vi "main.vi"() -> ()   [LabVIEW 2023]
uses:
  Controls/insutrument_data.ctl
  Controls/table_data.ctl
  <vilib>/Utility/error.llb/DialogType.ctl
  Controls/errors_type.ctl
panel:
  out "Description":string
  out "Time":string
  out "Error Code":string
  out "Type":T1
  out "Table 2":string[][](table)
  in  "stop 2":bool
  out "Waveform Chart 2":i32(graph)
  out "PSRR (dB) 2":i32
  in  "Eror log":bool
  out "Error?":bool
  in  "Wait time (sec)":i32=1 step=1
  out "error out":errorcluster
  in  "error in":errorcluster
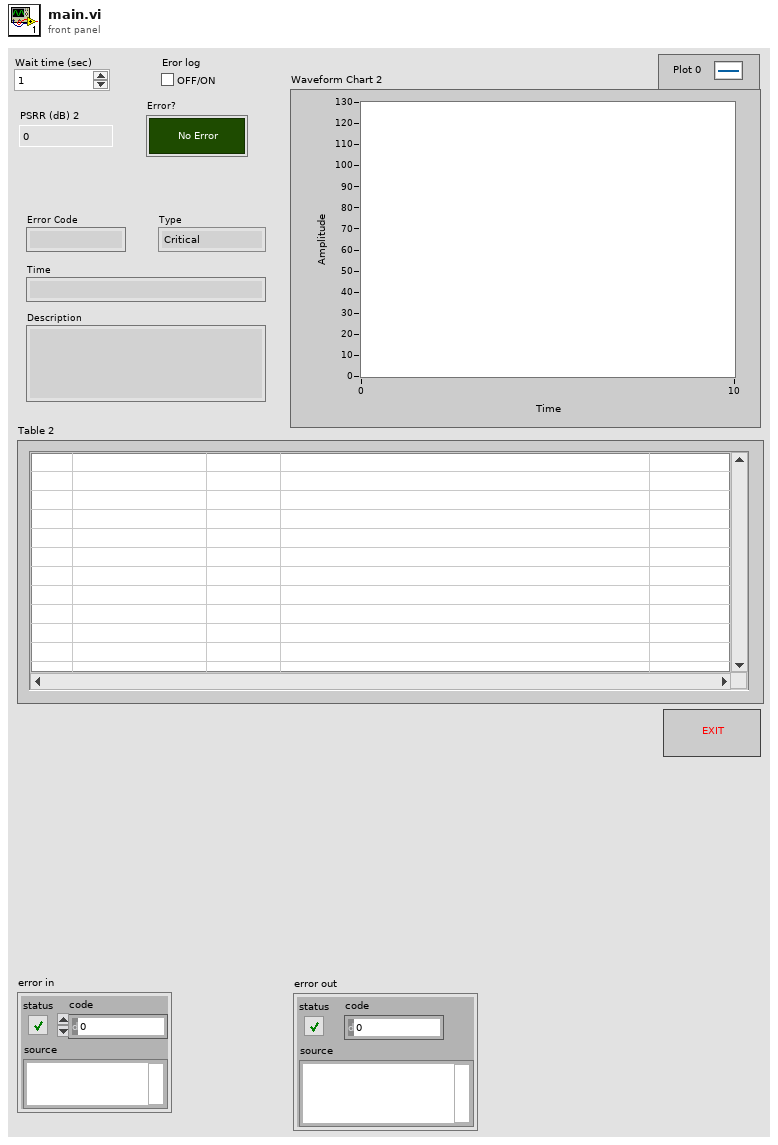
[diagram p1: front panel]
types:
  T1 = typedef "errors_type.ctl" = enum16{"Critical", "No error", "Warning", "Passive", "Unknown"}
  T2 = typedef "table_data.ctl" = cluster{"Passive_err":i32, "Unkown_err":i32, "Table_data":T3[][], "Err_log_sn":i32}
  T3 = typedef "insutrument_data.ctl" = string
  T4 = cluster{"Error Code":string, "Time":string, "Description":string, "Type":T1}
  T5 = typedef "DialogType.ctl" = u16
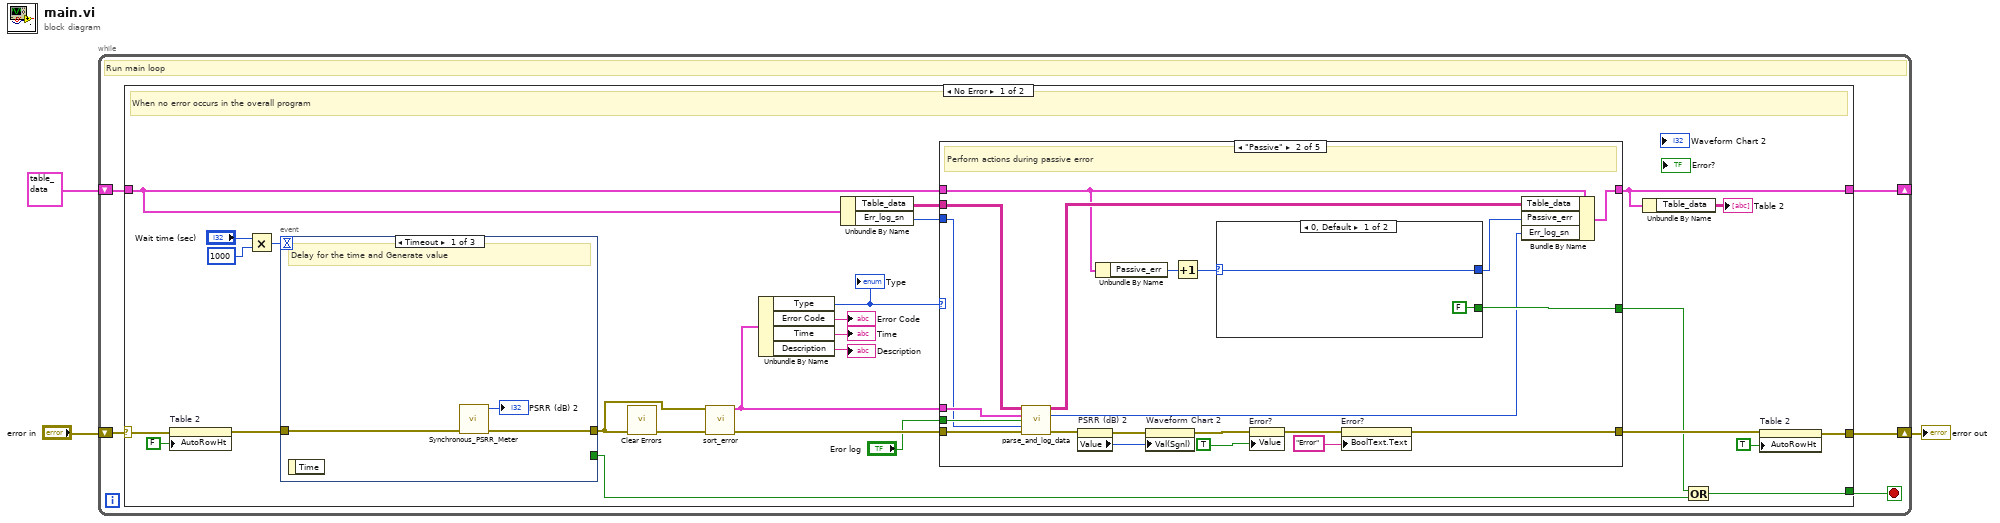
[diagram p0: block diagram]
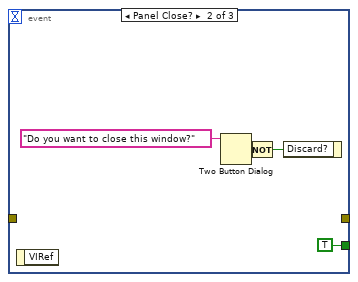
[diagram p2: hidden frame]
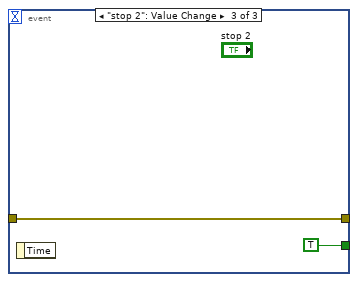
[diagram p3: hidden frame]
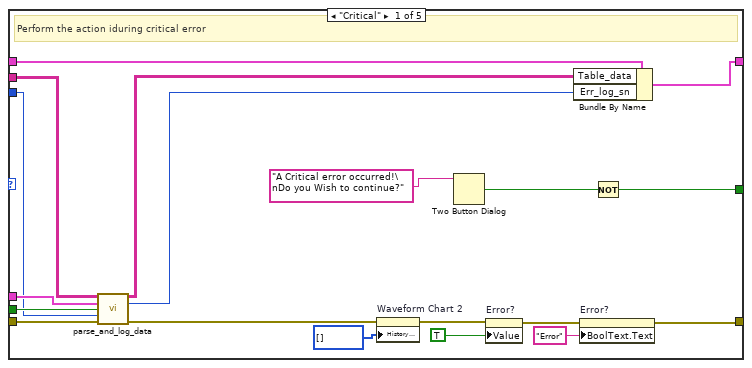
[diagram p4: hidden frame]
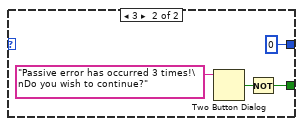
[diagram p5: hidden frame]
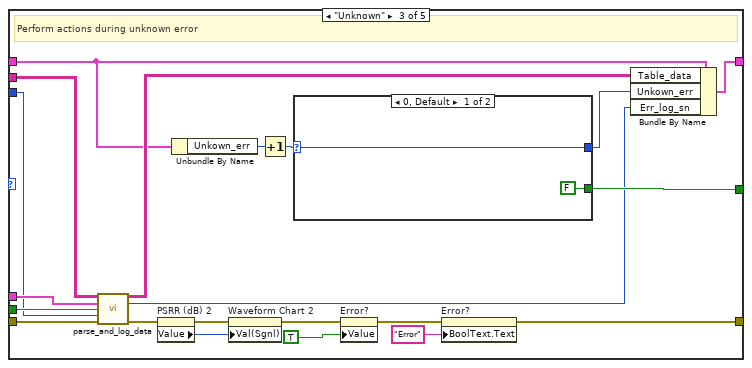
[diagram p6: hidden frame]
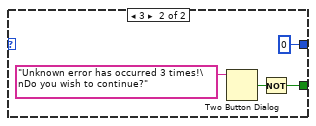
[diagram p7: hidden frame]
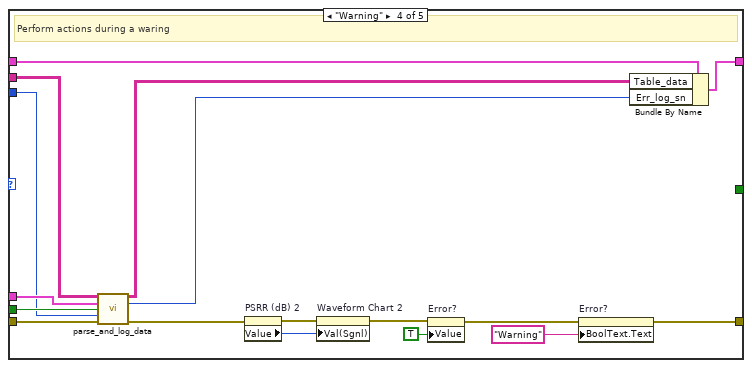
[diagram p8: hidden frame]
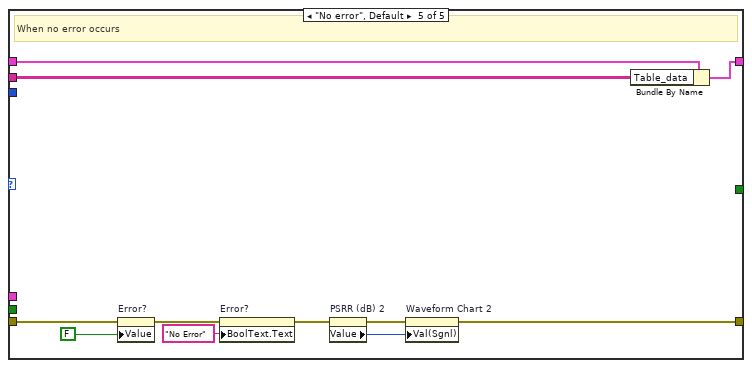
[diagram p9: hidden frame]
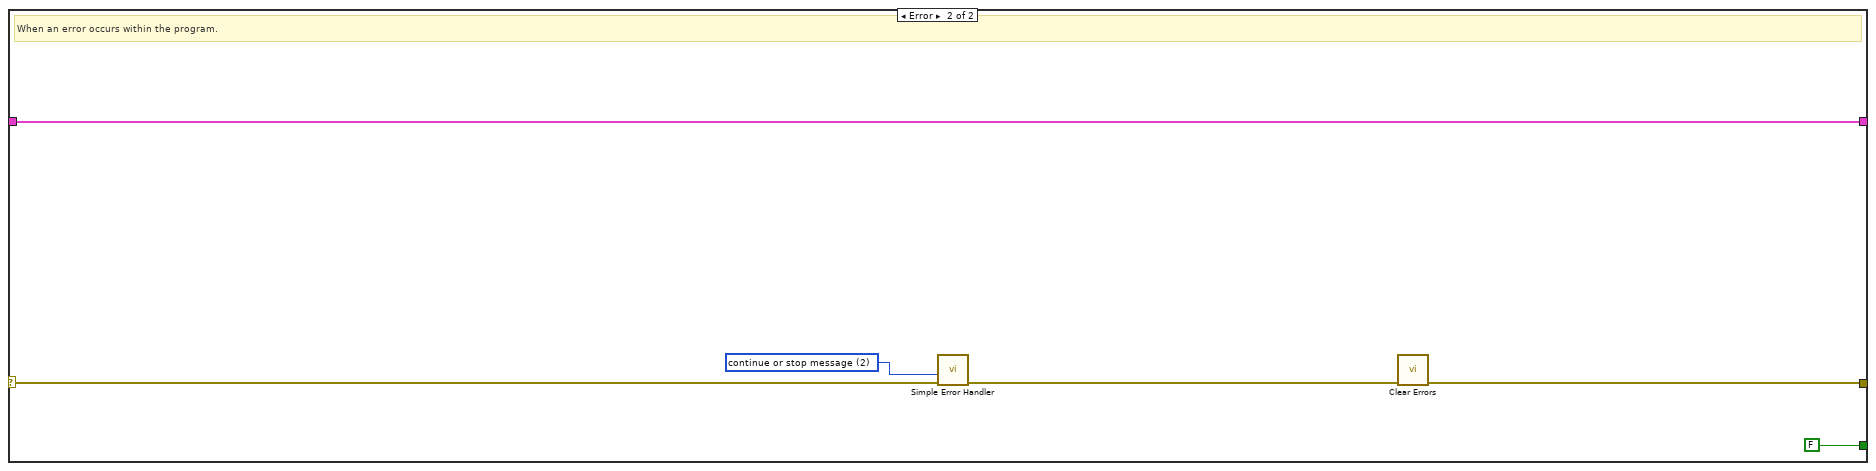
[diagram p10: hidden frame]
diagram:
  n1 = while {
    shift-right: [w7] -> w2
    shift-left: "error in" -> [w6]
    shift-right: [w4] -> _
    shift-left: T2 {"Passive_err"=0, "Unkown_err"=0, "Table_data"=[["SI No.", "Time of Occurenece", "Error Code", "Description", "Type"]], "Err_log_sn"=0} -> [w8]
    stop <- w5 stop-if-true
    # "Run main loop"
    n2 = case shown="No Error" w6 {
      selector: w6 -> [w22 w149]
      tunnel: w8 -> [w28 w150]
      tunnel: [w23 w145] -> w7
      tunnel: [w16 FALSE] -> w5
      tunnel: [w13 w150] -> w4
      frame No Error {
        # "When no error occurs in the overall program"
        n3 = property on="Table 2" class="Tbl (strict)"(error in=w22, "AutoRowHt"=FALSE ("Autosizing Row Height")) -> (error out=w21:errorcluster)  [unwired: 1 in, 1 out]
        n4 = Multiply(x="Wait time (sec)", y=1000) -> (x*y=w32:i32)
        n5 = event shown="[0] Timeout" {
          selector: _ -> [_ _ _]
          dyn-events: _ -> [_ _ _]
          timeout: w32 -> [_ _ _]
          tunnel: w21 -> [w37 _ w42]
          tunnel: [w36 _ w42] -> w31
          tunnel: [_ TRUE ("stop") TRUE ("stop")] -> w15
          event Timeout {
            # "Delay for the time and Generate value"
            n6 = event-data() -> ()  [unwired: 1 in, 1 out]
            n7 = call "Synchronous_PSRR_Meter.vi"("error in"=w37) -> ("error out"=w36:errorcluster, "PSRR (dB)"=→"PSRR (dB) 2":i32)  [unwired: 9 in]
          }
          event Panel Close? {
            n8 = event-data() -> ()  [unwired: 1 in, 1 out]
            n9 = Two Button Dialog(message="Do you want to close this window?") -> (T button?=w40:bool)  [unwired: 2 in]
            n10 = Not(x=w40) -> (.not. x?=w39:bool)
            n11 = event-data("Discard?"=w39) -> ()  [unwired: 1 in, 1 out]
          }
          event "stop 2": Value Change {
            n12 = event-data() -> ()  [unwired: 1 in, 1 out]
          }
        }
        n13 = call <vilib>:"Clear Errors.vi"("error in (no error)"=w31) -> ("error out"=w30:errorcluster)  [unwired: 5 in, 1 out]
        n14 = call "sort_error.vi"("check_error"=w31, "error constant"=w30) -> ("output cluster"=w27:T4, "error out"=w26:errorcluster)  [unwired: 12 in]
        n15 = Unbundle By Name(w27) -> ("Type"=w29:T1, "Error Code"=→"Error Code":string, "Time"=→"Time":string, "Description"=→"Description":string)
        "Type" <- w29
        n16 = Unbundle By Name(w28) -> ("Table_data"=w11:T3[][], "Err_log_sn"=w9:i32)
        n17 = case shown="\"Passive\"" w29 {
          tunnel: w28 -> [w49 w70 w97 w121 w135]
          tunnel: w27 -> [w62 w83 w110 w133 _]
          tunnel: w26 -> [w61 w82 w109 w132 w138]
          tunnel: [w54 w75 w102 w129 w142] -> w24
          tunnel: [w51 w66 w93 _ _] -> w14
          tunnel: [w47 w72 w99 w122 w136] -> w13
          tunnel: w11 -> [w50 w71 w98 w123 w134]
          tunnel: "Eror log" -> [w46 w65 w92 w119 _]
          tunnel: w9 -> [w45 w64 w91 w118 _]
          frame "Critical" {
            # "Perform the action iduring critical error"
            n18 = call "parse_and_log_data.vi"("Array"=w50, "Cluster"=w62, "file_log"=w46, "log_num"=w45, "error in"=w61) -> ("Table 2"=w48:string[][], "Num_out"=w44:i32, "error out"=w59:errorcluster)  [unwired: 8 in]
            n19 = property on="Waveform Chart 2" class="WFChart (strict)"(error in=w59, "History Data"=i32[] []) -> (error out=w55:errorcluster)  [unwired: 1 in, 1 out]
            n20 = Two Button Dialog(message="A Critical error occurred!\nDo you Wish to continue?") -> (T button?=w52:bool)  [unwired: 2 in]
            n21 = property on="Error?" class="Bool (strict)"(error in=w55, "Value"=TRUE ("Error?")) -> (error out=w58:errorcluster)  [unwired: 1 in, 1 out]
            n22 = Bundle By Name(cluster=w49, "Table_data"=w48, "Err_log_sn"=w44) -> (w47:T2)
            n23 = property on="Error?" class="Bool (strict)"(error in=w58, "BoolText.Text"="Error" ("Boolean Text.Text")) -> (error out=w54:errorcluster)  [unwired: 1 in, 1 out]
            n24 = Not(x=w52) -> (.not. x?=w51:bool)
          }
          frame "Passive" {
            # "Perform actions during passive error"
            n25 = call "parse_and_log_data.vi"("Array"=w71, "Cluster"=w83, "file_log"=w65, "log_num"=w64, "error in"=w82) -> ("Table 2"=w73:string[][], "Num_out"=w63:i32, "error out"=w79:errorcluster)  [unwired: 8 in]
            n26 = property on="PSRR (dB) 2" class="DigNum (strict)"(error in=w79) -> (error out=w80:errorcluster, "Value"=w81:i32)  [unwired: 1 in, 1 out]
            n27 = Unbundle By Name(w70) -> ("Passive_err"=w69:i32)
            n28 = property on="Waveform Chart 2" class="WFChart (strict)"(error in=w80, "Val(Sgnl)"=w81) -> (error out=w74:errorcluster)  [unwired: 1 in, 1 out]
            n29 = Increment(x=w69) -> (x+1=w68:i32)
            n30 = case shown="0, Default" w68 {
              selector: w68 -> [w85 _]
              tunnel: [w85 0] -> w67
              tunnel: [FALSE w86] -> w66
              frame 0, Default {
              }
              frame 3 {
                n31 = Two Button Dialog(message="Passive error has occurred 3 times!\nDo you wish to continue?") -> (T button?=w87:bool)  [unwired: 2 in]
                n32 = Not(x=w87) -> (.not. x?=w86:bool)
              }
            }
            n33 = property on="Error?" class="Bool (strict)"(error in=w74, "Value"=TRUE ("Error?")) -> (error out=w78:errorcluster)  [unwired: 1 in, 1 out]
            n34 = property on="Error?" class="Bool (strict)"(error in=w78, "BoolText.Text"="Error" ("Boolean Text.Text")) -> (error out=w75:errorcluster)  [unwired: 1 in, 1 out]
            n35 = Bundle By Name(cluster=w70, "Table_data"=w73, "Passive_err"=w67, "Err_log_sn"=w63) -> (w72:T2)
          }
          frame "Unknown" {
            # "Perform actions during unknown error"
            n36 = call "parse_and_log_data.vi"("Array"=w98, "Cluster"=w110, "file_log"=w92, "log_num"=w91, "error in"=w109) -> ("Table 2"=w100:string[][], "Num_out"=w90:i32, "error out"=w106:errorcluster)  [unwired: 8 in]
            n37 = property on="PSRR (dB) 2" class="DigNum (strict)"(error in=w106) -> (error out=w107:errorcluster, "Value"=w108:i32)  [unwired: 1 in, 1 out]
            n38 = Unbundle By Name(w97) -> ("Unkown_err"=w96:i32)
            n39 = property on="Waveform Chart 2" class="WFChart (strict)"(error in=w107, "Val(Sgnl)"=w108) -> (error out=w101:errorcluster)  [unwired: 1 in, 1 out]
            n40 = Increment(x=w96) -> (x+1=w95:i32)
            n41 = case shown="0, Default" w95 {
              selector: w95 -> [w112 _]
              tunnel: [w112 0] -> w94
              tunnel: [FALSE w113] -> w93
              frame 0, Default {
              }
              frame 3 {
                n42 = Two Button Dialog(message="Unknown error has occurred 3 times!\nDo you wish to continue?") -> (T button?=w114:bool)  [unwired: 2 in]
                n43 = Not(x=w114) -> (.not. x?=w113:bool)
              }
            }
            n44 = property on="Error?" class="Bool (strict)"(error in=w101, "Value"=TRUE ("Error?")) -> (error out=w105:errorcluster)  [unwired: 1 in, 1 out]
            n45 = property on="Error?" class="Bool (strict)"(error in=w105, "BoolText.Text"="Error" ("Boolean Text.Text")) -> (error out=w102:errorcluster)  [unwired: 1 in, 1 out]
            n46 = Bundle By Name(cluster=w97, "Table_data"=w100, "Unkown_err"=w94, "Err_log_sn"=w90) -> (w99:T2)
          }
          frame "Warning" {
            # "Perform actions during a waring"
            n47 = call "parse_and_log_data.vi"("Array"=w123, "Cluster"=w133, "file_log"=w119, "log_num"=w118, "error in"=w132) -> ("Table 2"=w120:string[][], "Num_out"=w117:i32, "error out"=w125:errorcluster)  [unwired: 8 in]
            n48 = property on="PSRR (dB) 2" class="DigNum (strict)"(error in=w125) -> (error out=w126:errorcluster, "Value"=w127:i32)  [unwired: 1 in, 1 out]
            n49 = property on="Waveform Chart 2" class="WFChart (strict)"(error in=w126, "Val(Sgnl)"=w127) -> (error out=w124:errorcluster)  [unwired: 1 in, 1 out]
            n50 = property on="Error?" class="Bool (strict)"(error in=w124, "Value"=TRUE ("Error?")) -> (error out=w131:errorcluster)  [unwired: 1 in, 1 out]
            n51 = property on="Error?" class="Bool (strict)"(error in=w131, "BoolText.Text"="Warning" ("Boolean Text.Text")) -> (error out=w129:errorcluster)  [unwired: 1 in, 1 out]
            n52 = Bundle By Name(cluster=w121, "Table_data"=w120, "Err_log_sn"=w117) -> (w122:T2)
          }
          frame "No error", Default {
            # "When no error occurs"
            n53 = property on="Error?" class="Bool (strict)"(error in=w138, "Value"=FALSE ("Error?")) -> (error out=w141:errorcluster)  [unwired: 1 in, 1 out]
            n54 = property on="Error?" class="Bool (strict)"(error in=w141, "BoolText.Text"="No Error" ("Boolean Text.Text")) -> (error out=w137:errorcluster)  [unwired: 1 in, 1 out]
            n55 = property on="PSRR (dB) 2" class="DigNum (strict)"(error in=w137) -> (error out=w143:errorcluster, "Value"=w144:i32)  [unwired: 1 in, 1 out]
            n56 = property on="Waveform Chart 2" class="WFChart (strict)"(error in=w143, "Val(Sgnl)"=w144) -> (error out=w142:errorcluster)  [unwired: 1 in, 1 out]
            n57 = Bundle By Name(cluster=w135, "Table_data"=w134) -> (w136:T2)
          }
        }
        n58 = Unbundle By Name(w13) -> ("Table_data"=→"Table 2":T3[][])
        n59 = Or(x=w14, y=w15) -> (x .or. y?=w16:bool)
        n60 = property on="Table 2" class="Tbl (strict)"(error in=w24, "AutoRowHt"=TRUE ("Autosizing Row Height")) -> (error out=w23:errorcluster)  [unwired: 1 in, 1 out]
      }
      frame Error {
        w146 = T5 2 items=["no dialog", "OK message", "continue or stop message", "OK message + warnings", "continue/stop + warnings"] ("type of dialog (OK msg:1)")
        # "When an error occurs within the program."
        n61 = call <vilib>:"Simple Error Handler.vi"("type of dialog (OK msg:1)"=w146, "error in (no error)"=w149) -> ("error out"=w147:errorcluster)  [unwired: 3 in, 4 out]
        n62 = call <vilib>:"Clear Errors.vi"("error in (no error)"=w147) -> ("error out"=w145:errorcluster)  [unwired: 5 in, 1 out]
      }
    }
  }
  "error out" <- w2
